vi "Voltage vs Signal_V1.vi"(6 "Maximum Deflection":dbl=3105.183 format="%#_13g", 7 "Maximum Voltage":dbl=264.0, 8 "b":dbl format="%#_13g", 9 "a":dbl format="%#_13g", 10 "Control Signal In (-1~1)":dbl[](array[numeric]), 11 "Voltage in (0~Max. Vol.)":dbl[](array[numeric])) -> (2 "Voltage Out (0~Max. Vol.)":dbl[](array[numeric]), 3 "Control Signal Out (-1~1)":dbl[](array[numeric]))   [LabVIEW 2014]
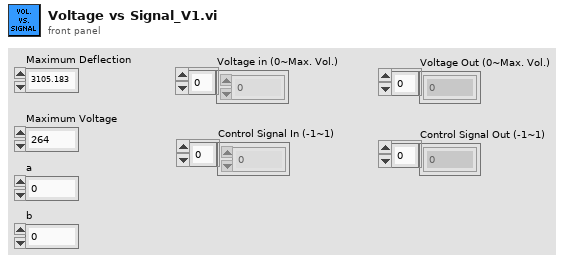
[diagram p1: front panel]
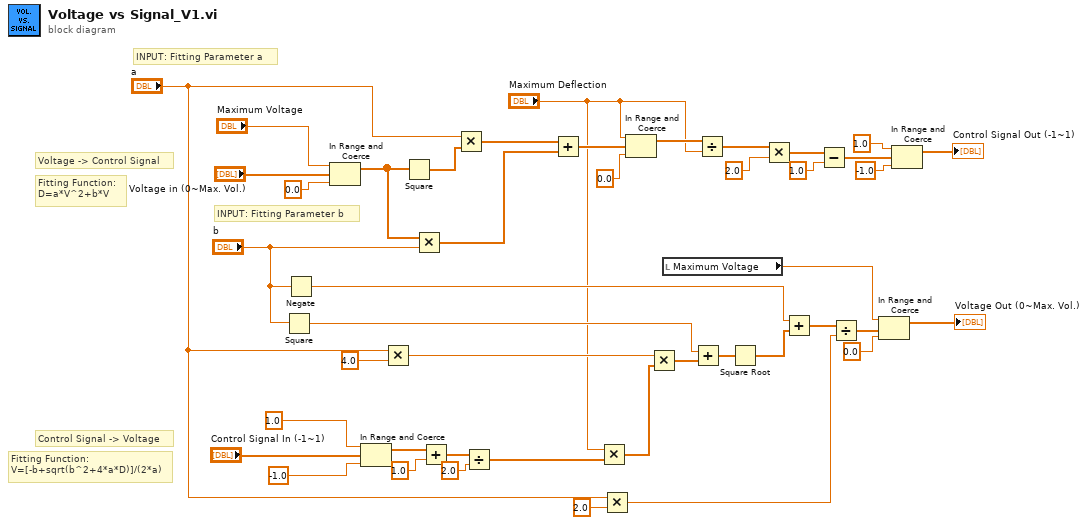
[diagram p0: block diagram]
diagram:
  # "Fitting Function:\nV=[-b+sqrt(b^2+4*a*D)]/(2*a)"
  # "Fitting Function:\nD=a*V^2+b*V"
  # "Control Signal -> Voltage"
  # "Voltage -> Control Signal"
  # "INPUT: Fitting Parameter b"
  # "INPUT: Fitting Parameter a"
  n1 = Square(x="b") -> (x^2=w20:dbl)
  n2 = Negate(x="b") -> (-x=w16:dbl)
  n3 = In Range and Coerce(upper limit="Maximum Voltage", x="Voltage in (0~Max. Vol.)", lower limit=0.0) -> (coerced(x)=w40:dbl[])  [unwired: 1 out]
  n4 = In Range and Coerce(upper limit=1.0, x="Control Signal In (-1~1)", lower limit=-1.0) -> (coerced(x)=w11:dbl[])  [unwired: 1 out]
  n5 = Multiply(x="a", y=4.0) -> (x*y=w25:dbl)
  n6 = Square(x=w40) -> (x^2=w44:dbl[])
  n7 = Multiply(x=w40, y="b") -> (x*y=w42:dbl[])
  n8 = Add(x=w11, y=1.0) -> (x+y=w9:dbl[])
  n9 = Multiply(x="a", y=w44) -> (x*y=w43:dbl[])
  n10 = Divide(x=w9, y=2.0) -> (x/y=w7:dbl[])
  n11 = Add(x=w43, y=w42) -> (x+y=w37:dbl[])
  n12 = Multiply(x="Maximum Deflection", y=w7) -> (x*y=w6:dbl[])
  n13 = Multiply(x="a", y=2.0) -> (x*y=w12:dbl)
  n14 = In Range and Coerce(upper limit="Maximum Deflection", x=w37, lower limit=0.0) -> (coerced(x)=w35:dbl[])  [unwired: 1 out]
  n15 = Multiply(x=w25, y=w6) -> (x*y=w21:dbl[])
  n16 = local read "Maximum Voltage"() -> (w3:dbl)
  n17 = Add(x=w20, y=w21) -> (x+y=w19:dbl[])
  n18 = Divide(x=w35, y="Maximum Deflection") -> (x/y=w34:dbl[])
  n19 = Square Root(x=w19) -> (sqrt(x)=w18:dbl[])
  n20 = Multiply(x=w34, y=2.0) -> (x*y=w32:dbl[])
  n21 = Add(x=w16, y=w18) -> (x+y=w15:dbl[])
  n22 = Subtract(x=w32, y=1.0) -> (x-y=w30:dbl[])
  n23 = Divide(x=w15, y=w12) -> (x/y=w5:dbl[])
  n24 = In Range and Coerce(upper limit=w3, x=w5, lower limit=0.0) -> (coerced(x)=→"Voltage Out (0~Max. Vol.)":dbl[])  [unwired: 1 out]
  n25 = In Range and Coerce(upper limit=1.0, x=w30, lower limit=-1.0) -> (coerced(x)=→"Control Signal Out (-1~1)":dbl[])  [unwired: 1 out]
